vi "上升沿检测.vi"(8 "error in":errorcluster, 11 "input":bool) -> (0 "error out":errorcluster, 3 "output":bool)   [LabVIEW 2017, in "边沿检测.lvlib"]
uses:
  <vilib>/ptbypt/NI_PtbyPt.lvlib
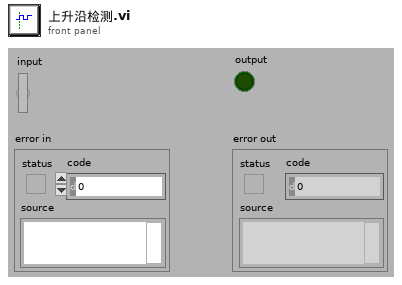
[diagram p1: front panel]
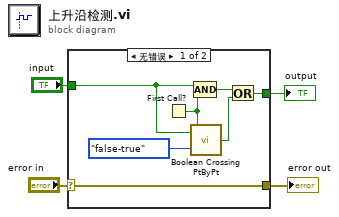
[diagram p0: block diagram]
diagram:
  n1 = case shown="无错误" "error in" {
    selector: "error in" -> [w10 w12]
    tunnel: "input" -> [w5 _]
    tunnel: [w8 _] -> w2
    tunnel: [w10 w12] -> w4
    frame No Error {
      n2 = First Call?() -> (First Call?: T/F=w6:bool)
      n3 = call <vilib>:"Boolean Crossing PtByPt.vi"("initialize"=w6, "direction"=enum16{"either", "false-true", "true-false"}."false-true", "input"=w5) -> ("crossing"=w7:bool)
      n4 = Compound Arithmetic op=AND(w5, w6) -> (w9:bool)
      n5 = Or(x=w9, y=w7) -> (x .or. y?=w8:bool)
    }
    frame Error {
    }
  }
  "output" <- w2
  "error out" <- w4
